vi "Google Earth - Test.vi"() -> ()   [LabVIEW 8.6]
panel:
  out "data":dbl[](array[numeric])
  in  "screen_y":dbl
  in  "screen_x":dbl
  out "Extents":T1
  in  "Set":bool
  in  "Set Camera Position":T2
  out "Camera Position":T2
  in  "stop":bool
  out "StreamingProgressPercentage":i32(slide) scale=0.0..100.0
  out "ElevationExaggeration":dbl
  out "AutoPilotSpeed":dbl
  out "VersionMinor":i32
  out "VersionMajor":i32
  out "VersionBuild":i32
  out "VersionAppType":i32(ring) items=["EnterpriseClientGE", "ProGE", "PlusGE", "FreeGE", "UnknownGE"]
  in  "error in":errorcluster
  in  "EARTHLib.IApplicationGE":refnum<k7>
  # "Lat"
  # "Lon"
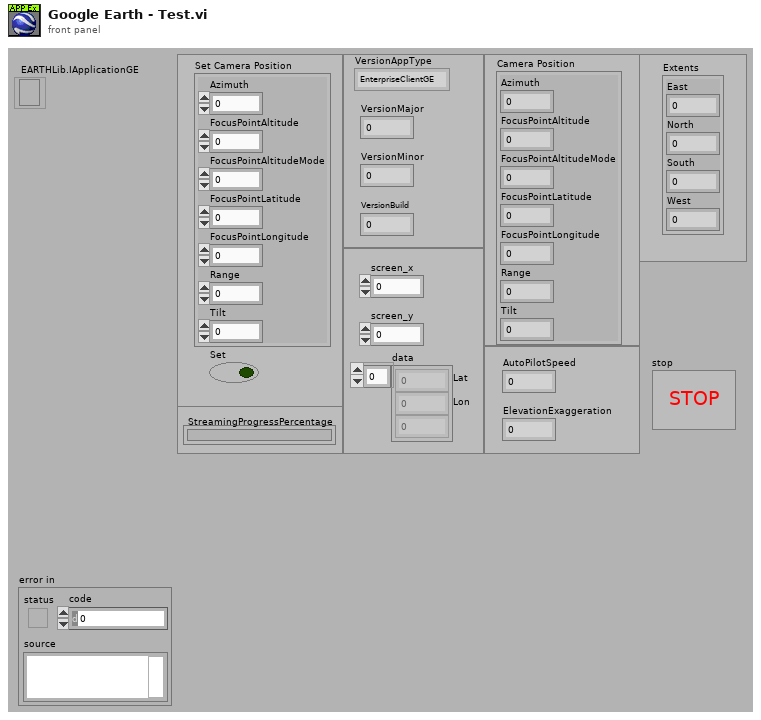
[diagram p1: front panel]
types:
  T1 = cluster{"East":dbl, "North":dbl, "South":dbl, "West":dbl}
  T2 = cluster{"Azimuth":dbl, "FocusPointAltitude":dbl, "FocusPointAltitudeMode":i32, "FocusPointLatitude":dbl, "FocusPointLongitude":dbl, "Range":dbl, "Tilt":dbl}
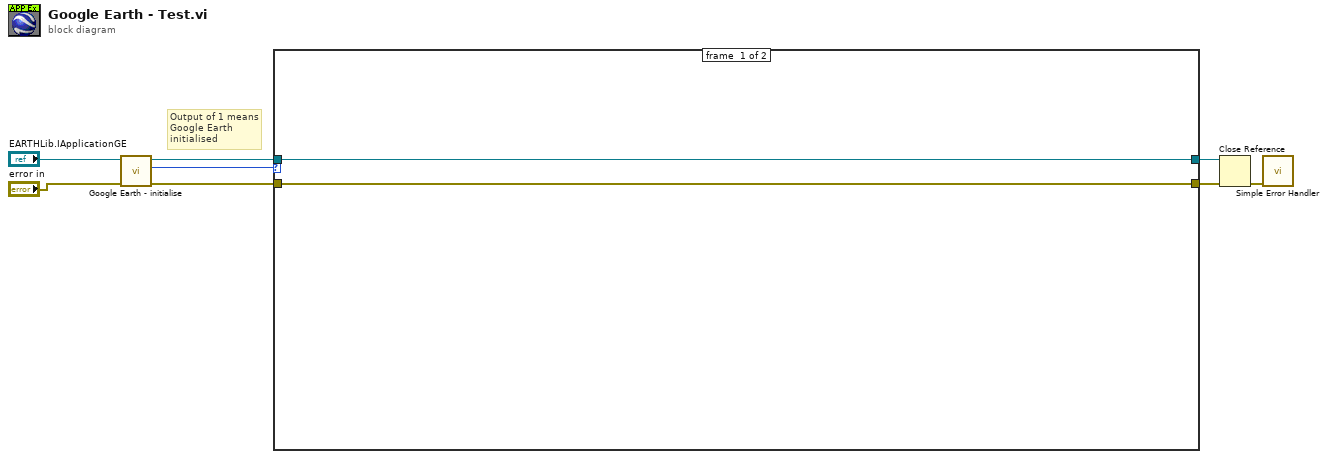
[diagram p0: block diagram]
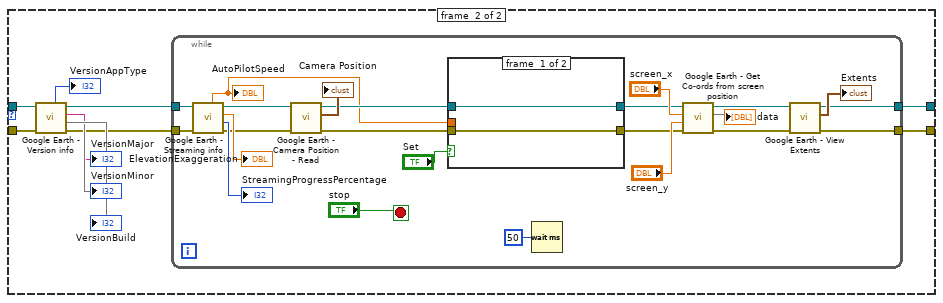
[diagram p2: hidden frame]
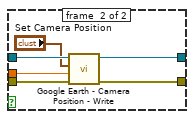
[diagram p3: hidden frame]
diagram:
  # "Output of 1 means\nGoogle Earth \ninitialised"
  n1 = call "Google Earth - initialise.vi"("error in (no error)"="error in", "EARTHLib.IApplicationGE"="EARTHLib.IApplicationGE") -> ("error out"=w6:errorcluster, "IsInitialized"=w7:i32, "Refnum Out"=w2:refnum<k7>)  [unwired: 7 in]
  n2 = case shown="1" w7 {
    tunnel: w2 -> [w9 w20]
    tunnel: w6 -> [w10 w19]
    tunnel: [w10 w12] -> w5
    tunnel: [w9 w11] -> w4
    frame #0 {
    }
    frame #1 {
      n3 = call "Google Earth - Version info.vi"("error in"=w19, "Refnum In"=w20) -> ("error out"=w14:errorcluster, 1:→"VersionMinor", "Version"=→"VersionMajor":string, "Refnum Out"=w13:refnum<k7>, 4:→"VersionBuild", "VersionAppType"=→"VersionAppType":i32)  [unwired: 4 in]
      n4 = while {
        tunnel: w13 -> [w43]
        tunnel: w14 -> [w42]
        tunnel: [w22] -> w12
        tunnel: [w25] -> w11
        stop <- "stop" stop-if-true
        n5 = call "Google Earth - Streaming info.vi"("error in"=w42, "Refnum in"=w43) -> ("error out"=w36:errorcluster, "StreamingProgressPercentage"=→"StreamingProgressPercentage":i32, "ElevationExaggeration"=→"ElevationExaggeration":dbl, "Refnum Out"=w37:refnum<k7>, "AutoPilotSpeed"=w33:dbl)  [unwired: 5 in]
        "AutoPilotSpeed" <- w33
        n6 = call "Google Earth - Camera Position - Read.vi"("error in"=w36, "Refnum in"=w37) -> ("error out"=w34:errorcluster, "Camera Position"=→"Camera Position":T2, "Refnum Out"=w35:refnum<k7>)  [unwired: 7 in]
        n7 = case shown="True" "Set" {
          tunnel: w35 -> [w44 w51]
          tunnel: w34 -> [w45 w50]
          tunnel: [w45 w49] -> w28
          tunnel: w33 -> [_ w47]
          tunnel: [w44 w46] -> w27
          frame #0 {
          }
          frame #1 {
            n8 = call "Google Earth - Camera Position - Write.vi"("error in"=w50, "speed"=w47, "Camera Position"="Set Camera Position", "Refnum in"=w51) -> ("error out"=w49:errorcluster, "Refnum Out"=w46:refnum<k7>)  [unwired: 6 in]
          }
        }
        n9 = Wait (ms)(milliseconds to wait=u32 50) -> ()  [unwired: 1 out]
        n10 = call "Google Earth - Get Co-ords from screen position.vi"("error in"=w28, "screen_y"="screen_y", "screen_x"="screen_x", "Refnum In"=w27) -> ("error out"=w23:errorcluster, 2:→"data", "RefnumOut"=w24:refnum<k7>)  [unwired: 5 in]
        n11 = call "Google Earth - View Extents.vi"("error in"=w23, "Refnum In"=w24) -> ("error out"=w22:errorcluster, "Extents"=→"Extents":T1, "Refnum Out"=w25:refnum<k7>)  [unwired: 7 in]
      }
    }
  }
  n12 = Close Reference(reference=w4, error in (no error)=w5) -> (error out=w1:errorcluster)
  n13 = call <vilib>:"Simple Error Handler.vi"("error in (no error)"=w1) -> ()  [unwired: 4 in, 5 out]
